vi "Heron's_Formula_for_Area_of_a_Triangle.vi"(2 "error in (no error)":errorcluster, 3 "c":dbl, 4 "b":dbl, 5 "a":dbl) -> (0 "error out":errorcluster, 1 "Pole trójkąta":dbl)   [LabVIEW 2021]
doc: "Program oblicza wzór Herona na pole trójkąta P = sqrt(p*(p-a)*(p-b)*(p-c))"
uses:
  <vilib>/Utility/error.llb/Error Cluster From Error Code.vi
  <vilib>/ErrorRing/Error Ring.xnode
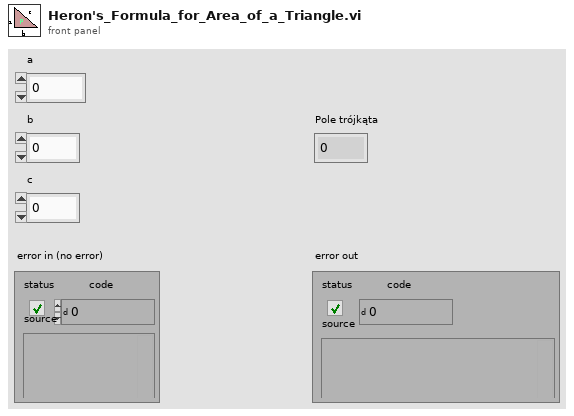
[diagram p1: front panel]
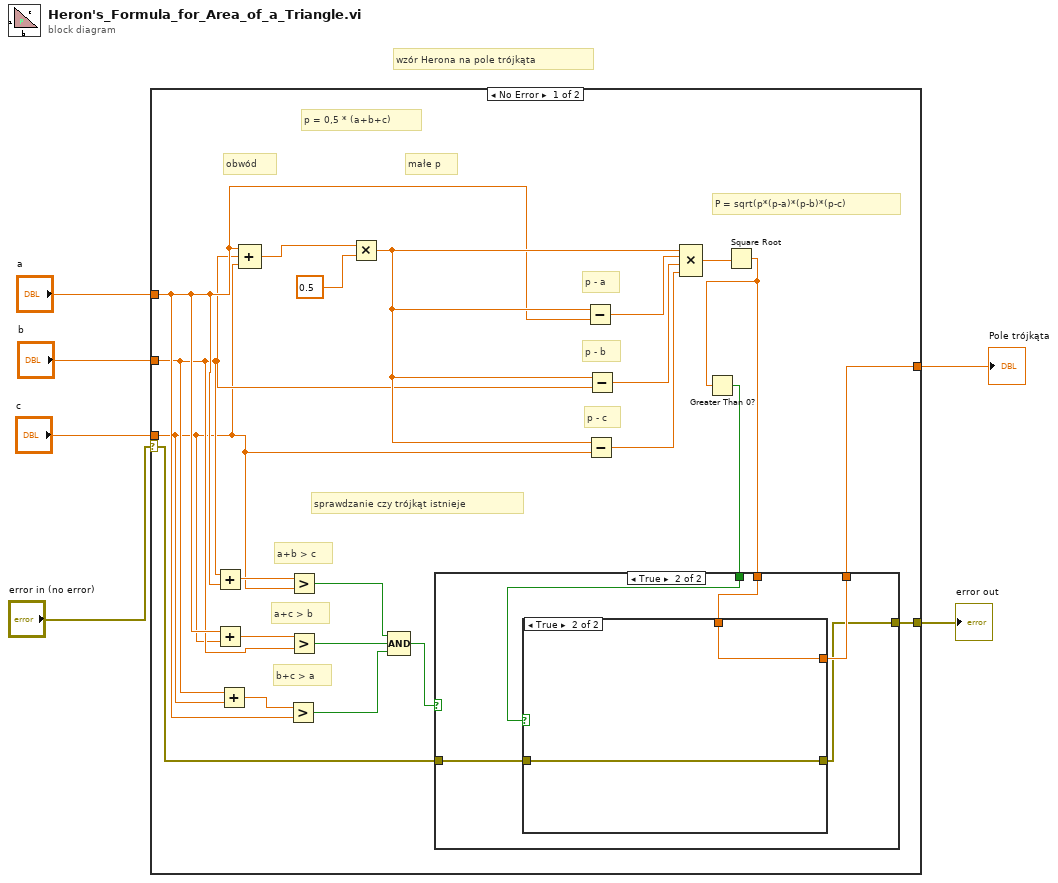
[diagram p0: block diagram]
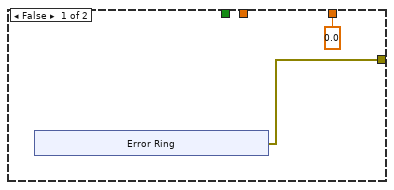
[diagram p2: hidden frame]
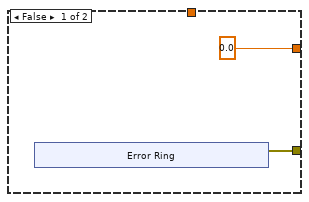
[diagram p3: hidden frame]
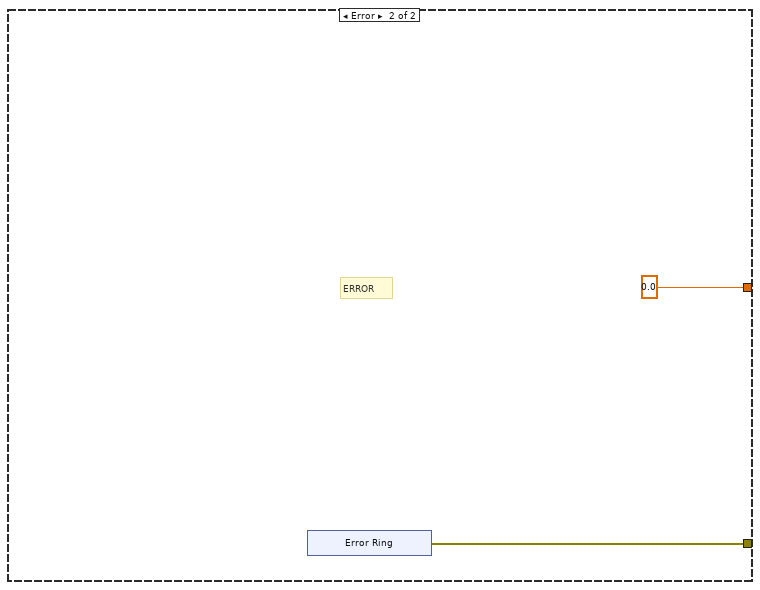
[diagram p4: hidden frame]
diagram:
  # "wzór Herona na pole trójkąta"
  n1 = case shown="No Error" "error in (no error)" {
    selector: "error in (no error)" -> [w20 _]
    tunnel: "a" -> [w13 _]
    tunnel: "b" -> [w12 _]
    tunnel: "c" -> [w11 _]
    tunnel: [w17 0.0] -> w3
    tunnel: [w21 w50] -> w1
    frame No Error {
      # "sprawdzanie czy trójkąt istnieje"
      # "a+b > c"
      # "a+c > b"
      # "b+c > a"
      # "p - c"
      # "p - b"
      # "p - a"
      # "P = sqrt(p*(p-a)*(p-b)*(p-c)"
      # "p = 0,5 * (a+b+c)"
      # "obwód"
      # "małe p"
      n2 = Add(x=w12, y=w13) -> (x+y=w14:dbl)
      n3 = Add(x=w13, y=w11) -> (x+y=w15:dbl)
      n4 = Add(x=w12, y=w11) -> (x+y=w16:dbl)
      n5 = Compound Arithmetic op=ADD(w13, w12, w11) -> (w27:dbl)
      n6 = Greater?(x=w16, y=w13) -> (0:w8:bool)
      n7 = Greater?(x=w14, y=w11) -> (0:w10:bool)
      n8 = Greater?(x=w15, y=w12) -> (0:w9:bool)
      n9 = Multiply(x=w27, y=0.5) -> (x*y=w26:dbl)
      n10 = Compound Arithmetic op=AND(w10, w9, w8) -> (w7:bool)
      n11 = Subtract(x=w26, y=w13) -> (x-y=w25:dbl)
      n12 = Subtract(x=w26, y=w11) -> (x-y=w23:dbl)
      n13 = Subtract(x=w26, y=w12) -> (x-y=w24:dbl)
      n14 = Compound Arithmetic op=MULTIPLY(w26, w25, w24, w23) -> (w22:dbl)
      n15 = Square Root(x=w22) -> (sqrt(x)=w18:dbl)
      n16 = Greater Than 0?(x=w18) -> (x > 0?=w19:bool)
      n17 = case shown="True" w7 {
        tunnel: [0.0 w40] -> w17
        tunnel: [w30 w39] -> w21
        tunnel: w20 -> [_ w38]
        tunnel: w19 -> [_ w37]
        tunnel: w18 -> [_ w36]
        frame False {
          n18 = xnode "Error Ring"() -> ("error out"=w30:errorcluster)
        }
        frame True {
          n19 = case shown="True" w37 {
            tunnel: [0.0 w49] -> w40
            tunnel: w36 -> [_ w49]
            tunnel: [w41 w48] -> w39
            tunnel: w38 -> [_ w48]
            frame False {
              n20 = xnode "Error Ring"() -> ("error out"=w41:errorcluster)
            }
            frame True {
            }
          }
        }
      }
    }
    frame Error {
      # "ERROR"
      n21 = xnode "Error Ring"() -> ("error out"=w50:errorcluster)
    }
  }
  "Pole trójkąta" <- w3
  "error out" <- w1
